vi "Read JSON.vi"(8 "error in (no error)":errorcluster, 11 "CycloneDX JSON in":refnum<class "CycloneDX JSON.lvclass">) -> (0 "error out":errorcluster, 2 "JSON":string="{}", 3 "CycloneDX JSON out":refnum<class "CycloneDX JSON.lvclass">)   [LabVIEW 2017, in "LabVIEW CycloneDX SBOM.lvlib" / "CycloneDX JSON.lvclass"]
uses:
  CycloneDX JSON.lvclass
  CycloneDX JSON.lvclass/CycloneDX JSON.ctl
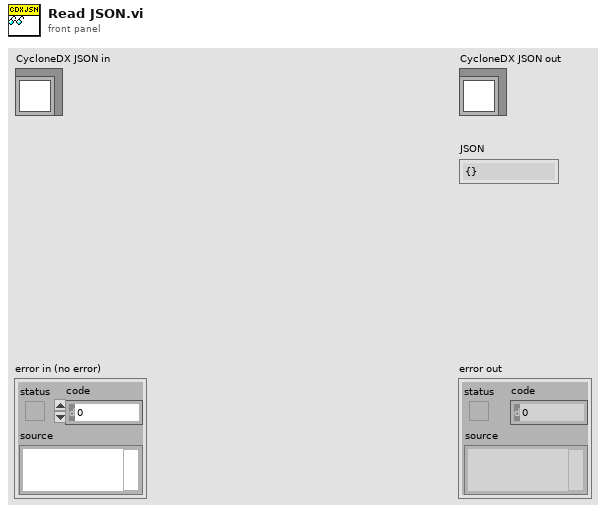
[diagram p1: front panel]
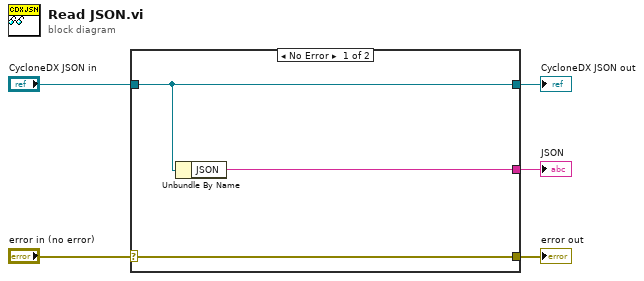
[diagram p0: block diagram]
diagram:
  n1 = case shown="No Error" "error in (no error)" {
    selector: "error in (no error)" -> [w8 w9]
    tunnel: [w8 w9] -> w4
    tunnel: [w7 w10] -> w2
    tunnel: "CycloneDX JSON in" -> [w7 w10]
    tunnel: [w6 _] -> w1
    frame No Error {
      n2 = Unbundle By Name(w7) -> ("JSON"=w6:string)
    }
    frame Error {
    }
  }
  "error out" <- w4
  "CycloneDX JSON out" <- w2
  "JSON" <- w1
